vi "apply modification.vi"(10 "vis":refnum<vi>[](array[refnum]), 11 "VI modification in":refnum<class "VI modification.lvclass">) -> (0 "error report":errorcluster[](array[cluster]), 3 "VI modification out":refnum<class "VI modification.lvclass">)   [LabVIEW 2013, in "VI modification.lvclass"]
uses:
  VI modification.lvclass
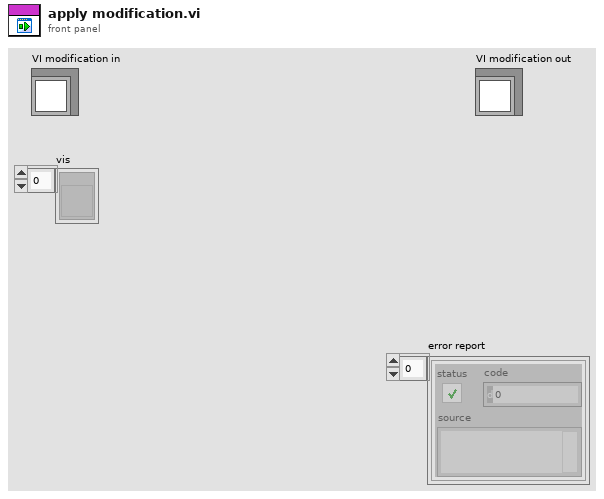
[diagram p1: front panel]
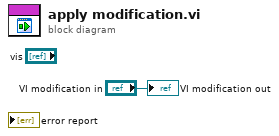
[diagram p0: block diagram]
diagram:
  "VI modification out" <- "VI modification in"
